vi "Pre Launch Init.vi"(11 "File Actor in":refnum<class "File Actor.lvclass">) -> (0 "error out":errorcluster, 3 "File Actor out":refnum<class "File Actor.lvclass">)   [LabVIEW 2018, in "File Library.lvlib" / "File Actor.lvclass"]
doc: "Retrieve file related information from the configuration file and open a new file."
uses:
  File Actor.lvclass
  C:/Program Files (x86)/National Instruments/LabVIEW 2018/vi.lib/MSR Consulting, LLC/General Reuse/SuperActor/SuperActor.lvclass
  <vilib>/MSR Consulting, LLC/General Reuse/Command/Command.lvclass
  <vilib>/MSR Consulting, LLC/General Reuse/SuperActor/SuperActor.lvclass/SuperActor.ctl
  File Actor.lvclass/File Actor.ctl
  <vilib>/MSR Consulting, LLC/General Reuse/SuperActor/Read Log Session.vi
  Messages/Abstract/Exe Write/Exe Write.lvclass
  C:/Program Files (x86)/National Instruments/LabVIEW 2018/vi.lib/MSR Consulting, LLC/General Reuse/Command/Command.lvclass
  <vilib>/MSR Consulting, LLC/General Reuse/SuperActor/SuperActor.lvclass
  <vilib>/MSR Consulting, LLC/General Reuse/Session APIs/_Session Fwk/Session - Root.lvclass
  <vilib>/MSR Consulting, LLC/General Reuse/Session APIs/Session Log/System Log.lvclass
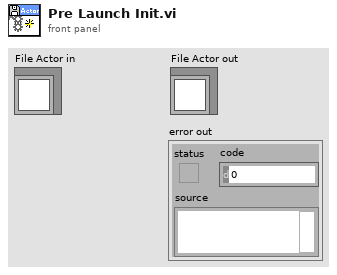
[diagram p1: front panel]
types:
  T1 = typedef "Session - Root.lvclass/Session Handle.ctl" = refnum<data-value>
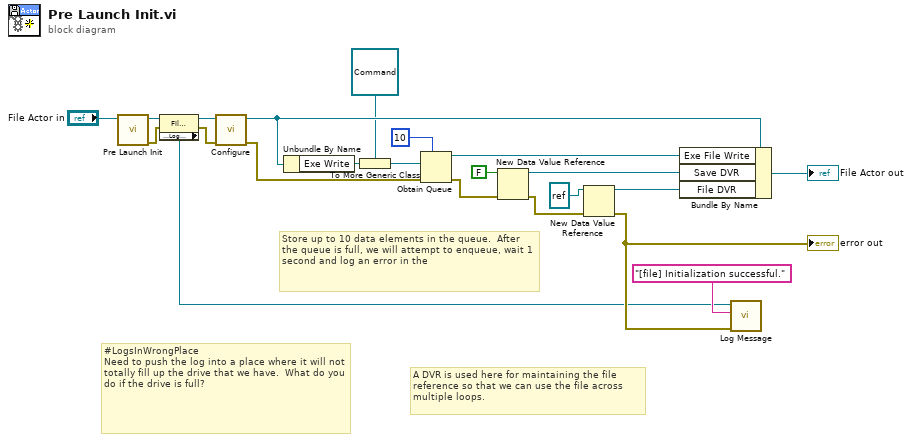
[diagram p0: block diagram]
diagram:
  # "#LogsInWrongPlace\nNeed to push the log into a place where it will not totally fill up the drive that we have.  What do you do if the drive is full?"
  # "Store up to 10 data elements in the queue.  After the queue is full, we will attempt to enqueue, wait 1 second and log an error in the"
  # "A DVR is used here for maintaining the file reference so that we can use the file across multiple loops."
  n1 = call-parent "Pre Launch Init.vi"("Ex Nested in"="File Actor in") -> ("error out"=w2:errorcluster, "Ex Nested out"=w5:refnum<class "File Actor.lvclass">)  [unwired: 9 in]
  n2 = property class="File Actor"(reference=w5, error in=w2) -> (reference out=w4:refnum<class "File Actor.lvclass">, error out=w1:errorcluster, "Accessors:Log Session"=w3:T1)
  n3 = call "Configure.vi"("error in"=w1, "File Actor in"=w4) -> ("error out"=w12:errorcluster, "File Actor out"=w18:refnum<class "File Actor.lvclass">)  [unwired: 8 in]
  n4 = Unbundle By Name(w18) -> ("Exe Write"=w16:refnum<class "Exe Write.lvclass">)
  n5 = To More Generic Class(target class=refnum<class "Command.lvclass"> refnum ("CMD"), reference=w16) -> (generic class reference=w14:refnum<class "Command.lvclass">)
  n6 = Obtain Queue(max queue size (-1, unlimited)=10, element data type=w14, error in (no error)=w12) -> (queue out=w13:refnum<queue>, error out=w10:errorcluster)  [unwired: 2 in, 1 out]
  n7 = New Data Value Reference(data value=FALSE, error in=w10) -> (data value reference=w7:refnum<data-value>, error out=w9:errorcluster)
  n8 = New Data Value Reference(data value=refnum<file> refnum ("File Ref"), error in=w9) -> (data value reference=w8:refnum<data-value>, error out=w19:errorcluster)
  "error out" <- w19
  n9 = Bundle By Name(cluster=w18, "Exe File Write"=w13, "Save DVR"=w7, "File DVR"=w8) -> (→"File Actor out":refnum<class "File Actor.lvclass">)
  n10 = call <vilib>:"Log Message.vi"("error in"=w19, "MSG In"="[file] Initialization successful.", "session in"=w3) -> ()  [unwired: 7 in, 2 out]
